vi "Setup Background BigMAQ.vi"(8 "error in":errorcluster, 9 "BigMAQ":refnum<class "BigMAQ.lvclass">, 10 "Display Settings":T1, 11 "Inset in":refnum<class "Inset.lvclass">) -> (0 "error out":errorcluster, 3 "Inset out":refnum<class "Inset.lvclass">)   [LabVIEW 2019, in "Inset.lvclass"]
uses:
  Inset.lvclass
  Inset.lvclass/Inset.ctl
  BigMAQ/BigMAQ.lvclass
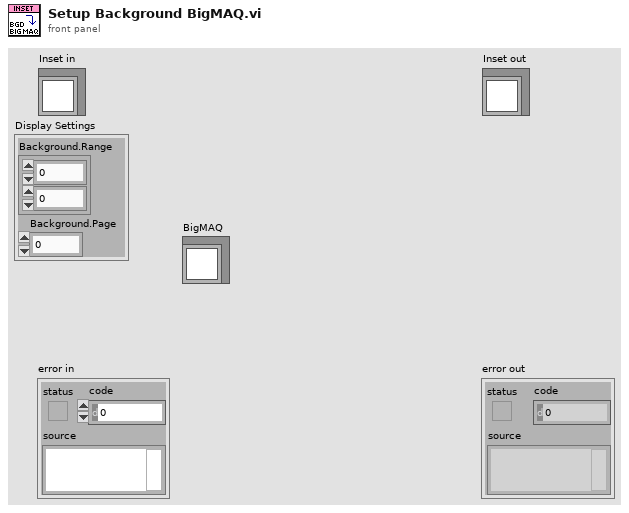
[diagram p1: front panel]
types:
  T1 = cluster{"Background.Range":cluster{sgl, sgl}, "Background.Page":i32}
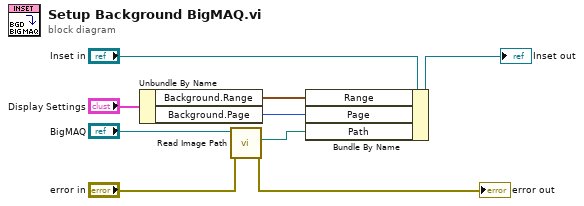
[diagram p0: block diagram]
diagram:
  n1 = Unbundle By Name("Display Settings") -> ("Background.Range"=w6:cluster{sgl, sgl}, "Background.Page"=w5:i32)
  n2 = call-dynamic "Read Image Path.vi"("error in (no error)"="error in", "BigMAQ in"="BigMAQ") -> ("error out"=→"error out":errorcluster, "Image Path"=w3:path)  [unwired: 7 in, 1 out]
  n3 = Bundle By Name(cluster="Inset in", "Range"=w6, "Page"=w5, "Path"=w3) -> (→"Inset out":refnum<class "Inset.lvclass">)
